vi "Untitled 7.vi"() -> ()   [LabVIEW 2021]
panel:
  out "Numeric":i32
  out "Százalékos eltérés":dbl
  out "Kimeneti feszültség":dbl
  in  "Feszültség":dbl
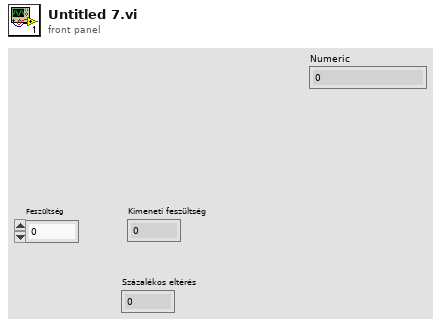
[diagram p1: front panel]
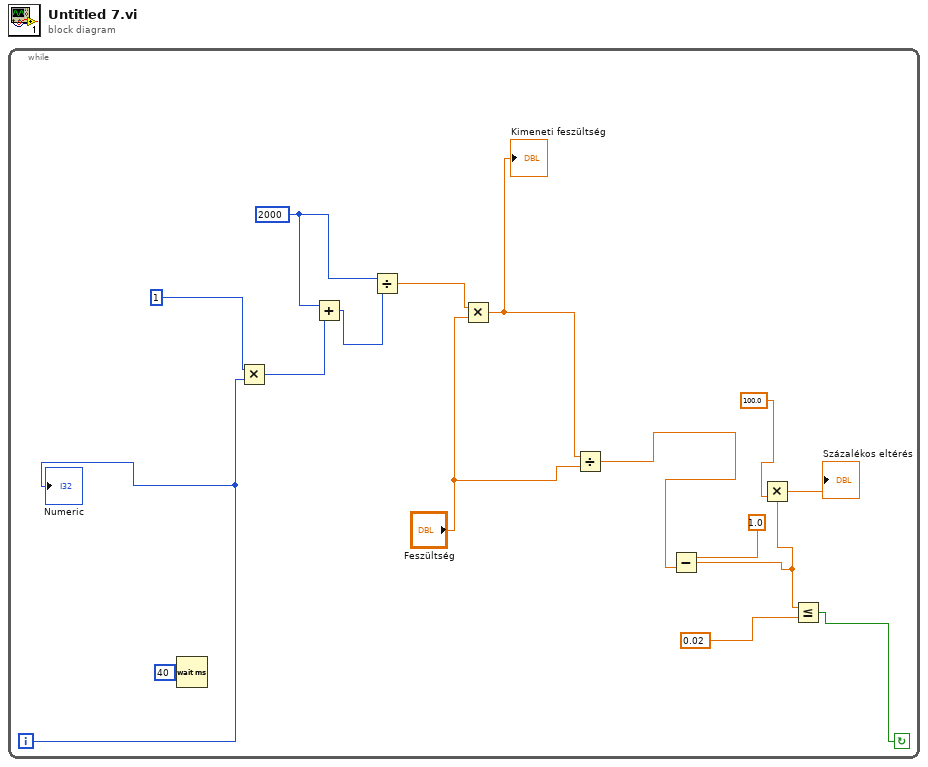
[diagram p0: block diagram]
diagram:
  n1 = while {
    i -> [w11]
    stop <- w8 continue-if-true
    w14 = 2000
    n2 = Wait (ms)(milliseconds to wait=u32 40) -> ()  [unwired: 1 out]
    n3 = Multiply(x=1, y=w11) -> (x*y=w13:i32)
    n4 = Add(x=w14, y=w13) -> (x+y=w12:i32)
    n5 = Divide(x=w14, y=w12) -> (x/y=w16:dbl)
    n6 = Multiply(x=w16, y="Feszültség") -> (x*y=w7:dbl)
    "Kimeneti feszültség" <- w7
    n7 = Divide(x=w7, y="Feszültség") -> (x/y=w4:dbl)
    n8 = Subtract(x=1.0, y=w4) -> (x-y=w2:dbl)
    n9 = Multiply(x=w2, y=100.0) -> (x*y=→"Százalékos eltérés":dbl)
    n10 = Less Or Equal?(x=w2, y=0.02 ("x")) -> (x <= y?=w8:bool)
    "Numeric" <- w11
  }
